vi "Read Sweep Sequence Configuration.vi"(8 "error in (no error)":errorcluster, 11 "Sweep Sequence in":refnum<class "Sweep.lvclass">) -> (0 "error out":errorcluster, 2 "Configuration":T1 {"Duration" format="%#_6ps"}, 3 "Sweep Sequence out":refnum<class "Sweep.lvclass">)   [LabVIEW 2018, in "Sweep.lvclass"]
uses:
  Sweep.lvclass
  C:/github/LabActor/Template Module/Template Module.lvclass
  Sweep Sequence Configuration.ctl
  Template Module/Template Module.lvclass/Template Module.ctl
  Template Module/Read Configuration.vi
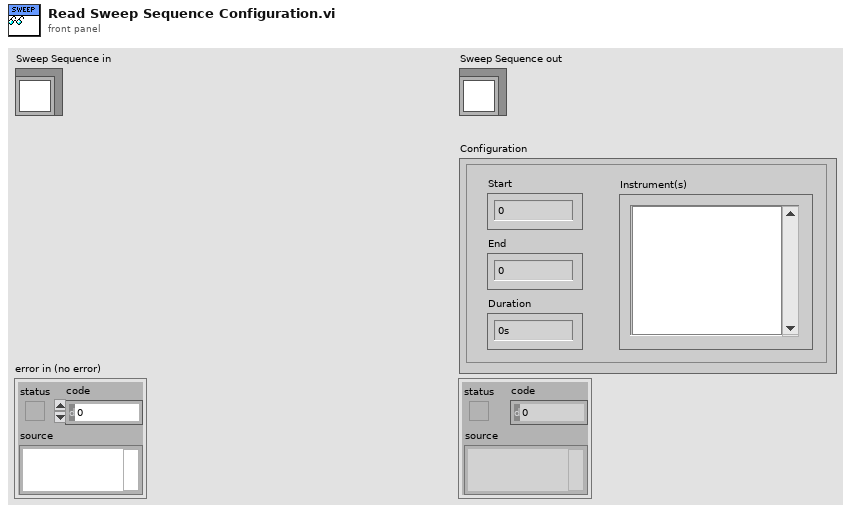
[diagram p1: front panel]
types:
  T1 = typedef "Sweep Sequence Configuration.ctl" = cluster{"Start":dbl, "End":dbl, "Duration":dbl, "Instrument(s)":i32}
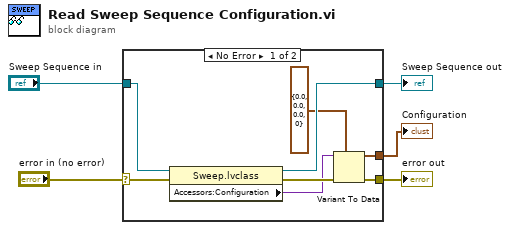
[diagram p0: block diagram]
diagram:
  n1 = case shown="No Error" "error in (no error)" {
    selector: "error in (no error)" -> [w13 w14]
    tunnel: [w9 w14] -> w4
    tunnel: [w10 w15] -> w2
    tunnel: "Sweep Sequence in" -> [w11 w15]
    tunnel: [w8 _] -> w1
    frame No Error {
      n2 = property class="Sweep.lvclass"(reference=w11, error in=w13) -> (reference out=w10:refnum<class "Sweep.lvclass">, error out=w12:errorcluster, "Accessors:Configuration"=w6:variant)
      n3 = Variant To Data(error in=w12, type=T1 {"Start"=0.0, "End"=0.0, "Duration"=0.0, "Instrument(s)"=0} ("Configuration"), Variant=w6) -> (data=w8:T1, error out=w9:errorcluster)
    }
    frame Error {
    }
  }
  "error out" <- w4
  "Sweep Sequence out" <- w2
  "Configuration" <- w1
